vi "new collection.vi"(8 "error in":errorcluster, 11 "tags":refnum<class "tag descriptor.lvclass">[](array[class])) -> (0 "error out":errorcluster, 3 "tag collection out":refnum<class "tag collection.lvclass">)   [LabVIEW 2013, in "tag bus.lvlib" / "tag collection.lvclass"]
uses:
  tag collection.lvclass
  tag/tag descriptor.lvclass
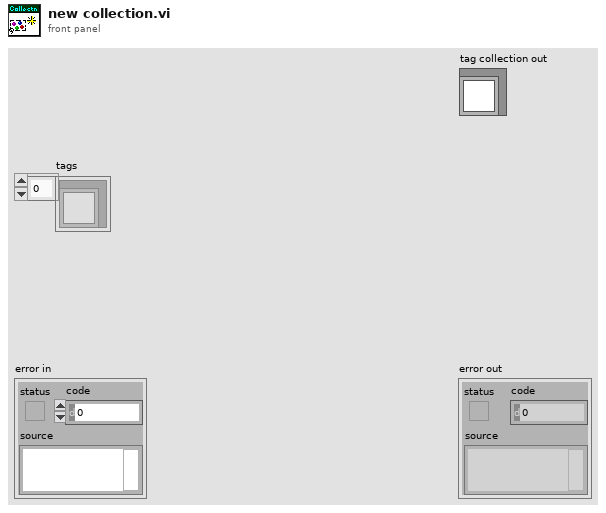
[diagram p1: front panel]
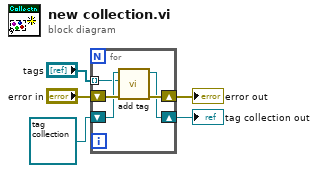
[diagram p0: block diagram]
diagram:
  n1 = for {
    shift-right: [w7] -> w2
    shift-left: refnum<class "tag collection.lvclass"> refnum ("tag collection in") -> [w8]
    shift-right: [w9] -> w4
    shift-left: "error in" -> [w10]
    tunnel: "tags" -> [w6] mode=indexing
    n2 = call "add tag.vi"("error in"=w10, "tag"=w6, "tag collection in"=w8) -> ("error out"=w9:errorcluster, "tag collection out"=w7:refnum<class "tag collection.lvclass">)  [unwired: 7 in]
  }
  "error out" <- w4
  "tag collection out" <- w2
